vi "APS pt enable.vi"(7 "AxisArr":i32, 8 "error in (no error)":errorcluster caption="错误输入（无错误）", 9 "Dimension":i32, 10 "PtbId":i32, 11 "Board_ID":i32) -> (0 "error out":errorcluster caption="错误输出", 3 "function return":i32, 5 "AxisArr out":i32)   [LabVIEW 2011, in "APS168.lvlib"]
doc: "I32 FNTYPE APS_pt_enable( I32 Board_ID, I32 PtbId, I32 Dimension, I32 *AxisArr );"
uses:
  APS168.lvlib
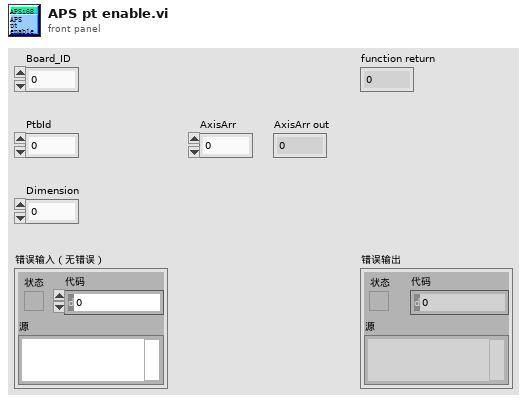
[diagram p1: front panel]
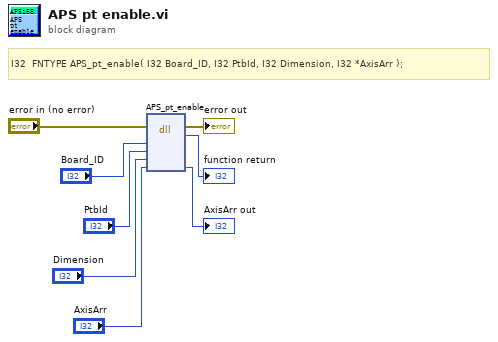
[diagram p0: block diagram]
diagram:
  # "I32  FNTYPE APS_pt_enable( I32 Board_ID, I32 PtbId, I32 Dimension, I32 *AxisArr );"
  n1 = dll-call lib="PTH1Labs E软件ADLINK 204CAPS_1_7_1_LIB line 连续运动204APS168.*" fn="APS_pt_enable"(error in="error in (no error)", "Board_ID"="Board_ID", "PtbId"="PtbId", "Dimension"="Dimension", "AxisArr"="AxisArr") -> (error out=→"error out":errorcluster, →"function return":i32, "AxisArr"=→"AxisArr out":i32)  [unwired: 5 in, 1 out]
